vi "AWG Get Timestamp.vi"(8 "error in (no error)":errorcluster, 11 "awg session in":T1={"type"=enum."Agilent 331xxA to 332xxA", "VISA"="", "enable 10MHz ref"=FALSE, "cmi ckd2"={"VISA"="", "clock source"=enum."Auto", "manual ref clk"=FALSE, "ref clock [Hz]"=0.0, "div mode"=enum."Set divisor directly"}, "cmi sync v3"={"VISA"="", "baud rate [bd/s]"=115200, "source"=enum."Auto", "hv range"=enum."1kV", "fsrc is fixed"=FALSE, "fsrc [Hz]"=10000000.0, "freq integ [s]"=1.0, "freq filter"=5, "trig level"=enum."TTL 5V", "chn1 mode"=enum."Source divider", "chn1 level"=enum."Positive 5V", "chn2 mode"=enum."Source divider", "chn2 level"=enum."Positive 5V", "chn2 div"=1, "chn3 mode"=enum."Chn 1 Active", "chn3 level"=enum."Positive 5V", "chn1 div entry"=enum."Calculate nearest divisor from measured fx", "chn1 dev limit [%]"=1.0, "chn1 check dev"=FALSE}, "trigger"={"source"=enum."Immediate", "level [V]"=0.0, "coupling"=enum."DC", "slope"=enum."POS"}, "HMF2500 cfg"={"Baud Rate"=9600, "Parity"=0, "Data Bits"=8, "Flow Control"=4}} {"HMF2500 cfg"."Flow Control" items=["None", "XON/XOFF", "RTS/CTS", "XON/XOFF & RTS/CTS", "DTR/DSR", "XON/XOFF & DTR/DSR"]; "HMF2500 cfg"."Data Bits" items=["7"=7, "8"=8]; "HMF2500 cfg"."Parity" items=["None", "Odd", "Even", "Mark", "Space"]; "HMF2500 cfg"."Baud Rate" items=["300"=300, "600"=600, "1200"=1200, "2400"=2400, "4800"=4800, "9600"=9600, "19200"=19200]; "cmi sync v3"."chn2 div" min=1 max=100000000 step=1; "cmi sync v3"."fsrc [Hz]" format="%_8p"}) -> (0 "error out":errorcluster, 2 "timestamp [s]":dbl, 3 "awg session out":T1={"type"=enum."Agilent 331xxA to 332xxA", "VISA"="", "enable 10MHz ref"=FALSE, "cmi ckd2"={"VISA"="", "clock source"=enum."Auto", "manual ref clk"=FALSE, "ref clock [Hz]"=0.0, "div mode"=enum."Set divisor directly"}, "cmi sync v3"={"VISA"="", "baud rate [bd/s]"=115200, "source"=enum."Auto", "hv range"=enum."1kV", "fsrc is fixed"=FALSE, "fsrc [Hz]"=10000000.0, "freq integ [s]"=1.0, "freq filter"=5, "trig level"=enum."TTL 5V", "chn1 mode"=enum."Source divider", "chn1 level"=enum."Positive 5V", "chn2 mode"=enum."Source divider", "chn2 level"=enum."Positive 5V", "chn2 div"=1, "chn3 mode"=enum."Chn 1 Active", "chn3 level"=enum."Positive 5V", "chn1 div entry"=enum."Calculate nearest divisor from measured fx", "chn1 dev limit [%]"=1.0, "chn1 check dev"=FALSE}, "trigger"={"source"=enum."Immediate", "level [V]"=0.0, "coupling"=enum."DC", "slope"=enum."POS"}, "HMF2500 cfg"={"Baud Rate"=9600, "Parity"=0, "Data Bits"=8, "Flow Control"=4}} {"HMF2500 cfg"."Flow Control" items=["None", "XON/XOFF", "RTS/CTS", "XON/XOFF & RTS/CTS", "DTR/DSR", "XON/XOFF & DTR/DSR"]; "HMF2500 cfg"."Data Bits" items=["7"=7, "8"=8]; "HMF2500 cfg"."Parity" items=["None", "Odd", "Even", "Mark", "Space"]; "HMF2500 cfg"."Baud Rate" items=["300"=300, "600"=600, "1200"=1200, "2400"=2400, "4800"=4800, "9600"=9600, "19200"=19200]; "cmi sync v3"."chn2 div" min=1 max=100000000 step=1; "cmi sync v3"."fsrc [Hz]" format="%_8p"})   [LabVIEW 2020, in "AWG.lvlib"]
doc: "AWG wrapper: Get last pulse train initial timestamp if supported."
uses:
  AWG.lvlib
  CMI Sync V3/CMI Sync Unit V3.lvlib
  AWG Type.ctl
  AWG Session.ctl
  CMI Clock Divider v2/CMI ckd2 Source Mode.ctl
  CMI Clock Divider v2/CMI ckd2 Session.ctl
  CMI Sync V3/Configure/CMI Sync V3 Reference Clock Source.ctl
  CMI Sync V3/Configure/CMI Sync V3 HV input Range.ctl
  CMI Sync V3/Configure/CMI Sync V3 Trigger Input Level.ctl
  CMI Sync V3/Configure/CMI Sync V3 Channel 1 Mode.ctl
  CMI Sync V3/Configure/CMI Sync V3 Channel Output Levels.ctl
  CMI Sync V3/Configure/CMI Sync V3 Channel 2 Mode.ctl
  CMI Sync V3/Configure/CMI Sync V3 Channel 3 Mode.ctl
  CMI Sync V3/CMI Sync V3 session.ctl
  CMI Clock Divider v2/CMI ckd2 Divisor Mode.ctl
  CMI Sync V3/Configure/CMI Sync V3 Channel 1 Divisor Entry Mode.ctl
  externals needed for AWG/ADC Trig Mode Source.ctl
  externals needed for AWG/ADC Trig Coupling.ctl
  externals needed for AWG/ADC Trig Slope.ctl
  externals needed for AWG/ADC Trig Config.ctl
  RaS HMF2500/HMF2500 Config.ctl
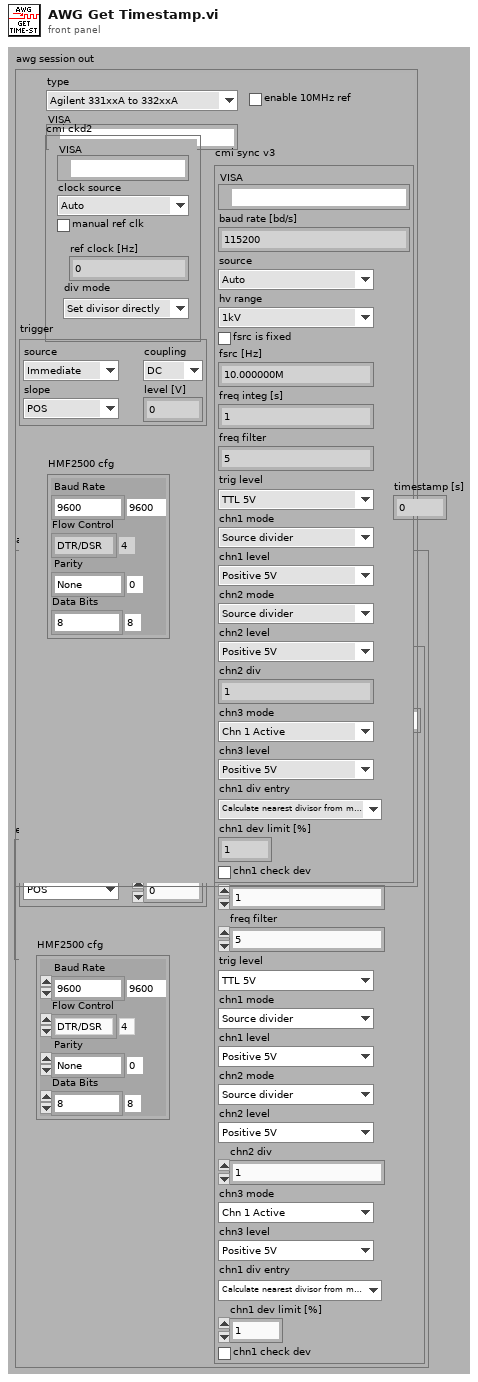
[diagram p1: front panel]
types:
  T1 = typedef "AWG.lvlib/AWG Session.ctl" = cluster{"type":T2, "VISA":refnum<visa-resource-name>, "enable 10MHz ref":bool, "cmi ckd2":T3, "cmi sync v3":T6, "trigger":T15, "HMF2500 cfg":T19}
  T2 = typedef "AWG.lvlib/AWG Type.ctl" = enum16{"Agilent 331xxA to 332xxA", "Agilent 335xxA to 336xxA", "Tektronix AFG3101C", "R&S HMF25xx", "CMI Clock Divider v2", "CMI Sync Unit V3", "dummy"}
  T3 = typedef "AWG.lvlib/CMI ckd2 Session.ctl" = cluster{"VISA":refnum<visa-resource-name>, "clock source":T4, "manual ref clk":bool, "ref clock [Hz]":dbl, "div mode":T5}
  T4 = typedef "AWG.lvlib/CMI ckd2 Source Mode.ctl" = enum16{"Auto", "LF clock", "HF clock", "Internal"}
  T5 = typedef "AWG.lvlib/CMI ckd2 Divisor Mode.ctl" = enum16{"Set divisor directly", "Set divisor by frequency"}
  T6 = typedef "AWG.lvlib/CMI Sync Unit V3.lvlib/CMI Sync V3 session.ctl" = cluster{"VISA":refnum<visa-resource-name>, "baud rate [bd/s]":i32, "source":T7, "hv range":T8, "fsrc is fixed":bool, "fsrc [Hz]":dbl, "freq integ [s]":dbl, "freq filter":i32, "trig level":T9, "chn1 mode":T10, "chn1 level":T11, "chn2 mode":T12, "chn2 level":T11, "chn2 div":i32, "chn3 mode":T13, "chn3 level":T11, "chn1 div entry":T14, "chn1 dev limit [%]":dbl, "chn1 check dev":bool}
  T7 = typedef "AWG.lvlib/CMI Sync Unit V3.lvlib/CMI Sync V3 Reference Clock Source.ctl" = enum16{"Auto", "Internal", "Logic", "Sine", "HV"}
  T8 = typedef "AWG.lvlib/CMI Sync Unit V3.lvlib/CMI Sync V3 HV input Range.ctl" = enum16{"10V", "60V", "250V", "1kV"}
  T9 = typedef "AWG.lvlib/CMI Sync Unit V3.lvlib/CMI Sync V3 Trigger Input Level.ctl" = enum16{"LVCMOS 3V3", "TTL 5V"}
  T10 = typedef "AWG.lvlib/CMI Sync Unit V3.lvlib/CMI Sync V3 Channel 1 Mode.ctl" = enum16{"Source divider", "DDS absolute", "DDS ratio", "DDS ratio M/N"}
  T11 = typedef "AWG.lvlib/CMI Sync Unit V3.lvlib/CMI Sync V3 Channel Output Levels.ctl" = enum16{"Positive 3V3", "Negative 3V3", "Positive 5V", "Negative 5V"}
  T12 = typedef "AWG.lvlib/CMI Sync Unit V3.lvlib/CMI Sync V3 Channel 2 Mode.ctl" = enum16{"Source divider", "Chn 1 divide"}
  T13 = typedef "AWG.lvlib/CMI Sync Unit V3.lvlib/CMI Sync V3 Channel 3 Mode.ctl" = enum16{"Chn 1 Active", "Chn 2 Active", "Chn 1 Trigger", "Chn 2 Trigger", "Gate", "PPS", "10MHz"}
  T14 = typedef "AWG.lvlib/CMI Sync Unit V3.lvlib/CMI Sync V3 Channel 1 Divisor Entry Mode.ctl" = enum16{"Set divisor directly", "Calculate nearest divisor from measured fx"}
  T15 = typedef "ADC Trig Config.ctl" = cluster{"source":T16, "level [V]":dbl, "coupling":T17, "slope":T18}
  T16 = typedef "ADC Trig Mode Source.ctl" = enum16{"Immediate", "External", "Level"}
  T17 = typedef "ADC Trig Coupling.ctl" = enum16{"DC", "AC"}
  T18 = typedef "ADC Trig Slope.ctl" = enum16{"POS", "NEG"}
  T19 = typedef "AWG.lvlib/HMF2500 Config.ctl" = cluster{"Baud Rate":u32, "Parity":u16, "Data Bits":u16, "Flow Control":u16}
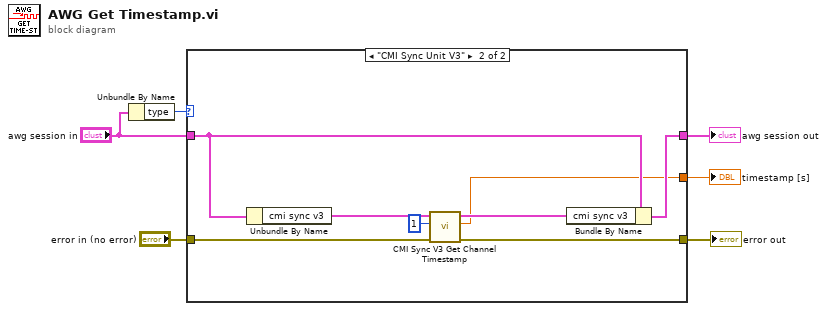
[diagram p0: block diagram]
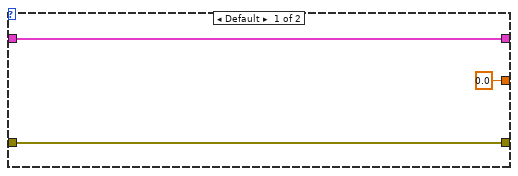
[diagram p2: hidden frame]
diagram:
  n1 = Unbundle By Name("awg session in") -> ("type"=w6:T2)
  n2 = case shown="\"CMI Sync Unit V3\"" w6 {
    tunnel: "error in (no error)" -> [w9 w15]
    tunnel: [w9 w14] -> w4
    tunnel: "awg session in" -> [w8 w17]
    tunnel: [w8 w16] -> w2
    tunnel: [0.0 ("timestamp [s]") w10] -> w1
    frame Default {
    }
    frame "CMI Sync Unit V3" {
      n3 = Unbundle By Name(w17) -> ("cmi sync v3"=w13:T6)
      n4 = call "CMI Sync V3 Get Channel Timestamp.vi"("error in"=w15, "Channel (1)"=1, "session in"=w13) -> ("error out"=w14:errorcluster, "timestamp [s]"=w10:dbl, "session out"=w12:T6)  [unwired: 6 in]
      n5 = Bundle By Name(cluster=w17, "cmi sync v3"=w12) -> (w16:T1)
    }
  }
  "error out" <- w4
  "awg session out" <- w2
  "timestamp [s]" <- w1
